vi "Show Cursors.vi"(6 "Cursor Options":T1={"font"={"Font Name"="Arial", "Size"=14, "Strikeout?"=FALSE, "Italic?"=FALSE, "Underline?"=FALSE, "Outline?"=FALSE, "Shadow?"=FALSE, "Bold?"=FALSE}, "size"=1, "Timestamp"=enum."at TOP", "Vertical Line?"=FALSE, "Horizontal Line?"=FALSE, "alignment(left, top)"={"horizontal"=enum."center", "vertical"=enum."center"}, "TextFormat"="%2$.2f\\n\\n%1$s", "time format (%H:%M:%S)"="Arial"} {"size" min=1 max=50}, 8 "error in (no error)":errorcluster, 9 "Coords":T2, 10 "XY Graph":refnum<vi>, 11 "input picture":picture) -> (0 "error out":errorcluster, 3 "output picture":picture)   [LabVIEW 2015]
doc: "Shows real time cursors overlayed in a graph, using just one mouse move event case. The options for the cursors can be highly customized to set up a unique cursor style.\n\nUsage: Place this inside an event structure on any XY graph, in the \"Mouse Move\" event case. Set the options as an input cluster to override the defaults. The output picture control would typically be connected to the XY Graph's \"PlotImages.Front\" property item.\n\nCursor Options\n<b>Horizontal Line?</b> - Draws a horizontal line to intersect each plot\n<b>Verticle Line?</b> - Draws a verticle line at the mouse location to highlight the cursor location (typically on the time scale)\n<b>Timestamp</b> - Sets where to display the timestamp (if you want it at the top or bottom) Used best with the verticle line turned on.\n<b>Font</b> - Setup the font for displaying the cursor text\n<b>Alignment</b> - Sets the alignment options for the text relative to the cursor point\n<b>TextFormat</b> - Sets the text display format at the cursor points to show. Three input parameters are available for the text, which can be accessed using parameter numbers.\ninputs: \n1$ - Timestamp at cursor locations\n2$ - Value of the plot\n3$ - Name of the plot\n\nExamples: $2$.2f\\n\\n%1$s\nThis shows the value of the plot with 2 decimal places. A blank line, then the name of the plot"
uses:
  <vilib>/Utility/miscctls.llb/LVPoint32TypeDef.ctl
  controls/CursorOptions.ctl
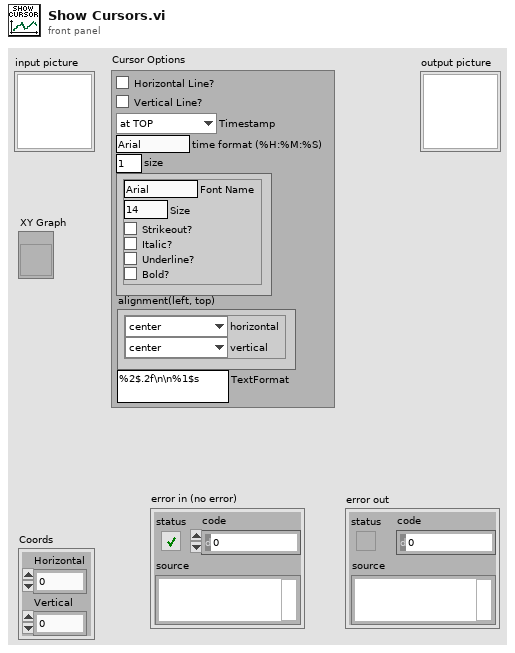
[diagram p1: front panel]
types:
  T1 = typedef "CursorOptions.ctl" = cluster{"font":cluster{"Font Name":string, "Size":i16, "Strikeout?":bool, "Italic?":bool, "Underline?":bool, "Outline?":bool, "Shadow?":bool, "Bold?":bool}, "size":i16, "Timestamp":enum16{"at TOP", "at BOTTOM", "none"}, "Vertical Line?":bool, "Horizontal Line?":bool, "alignment(left, top)":cluster{"horizontal":enum16{"left", "center", "right"}, "vertical":enum16{"top", "center", "bottom"}}, "TextFormat":string, "time format (%H:%M:%S)":string}
  T2 = typedef "LVPoint32TypeDef.ctl" = cluster{"Horizontal":i32, "Vertical":i32}
  T3 = enum16{"User-specified Font", "Application Font", "System Font", "Dialog Font"}
  T4 = cluster{"horizontal":enum16{"left", "center", "right"}, "vertical":enum16{"top", "center", "bottom"}}
  T5 = cluster{"Font Name":string, "Size":i16, "Strikeout?":bool, "Italic?":bool, "Underline?":bool, "Outline?":bool, "Shadow?":bool, "Bold?":bool}
  T6 = typedef "LVRectTypeDef.ctl" = cluster{"Left":i16, "Top":i16, "Right":i16, "Bottom":i16}
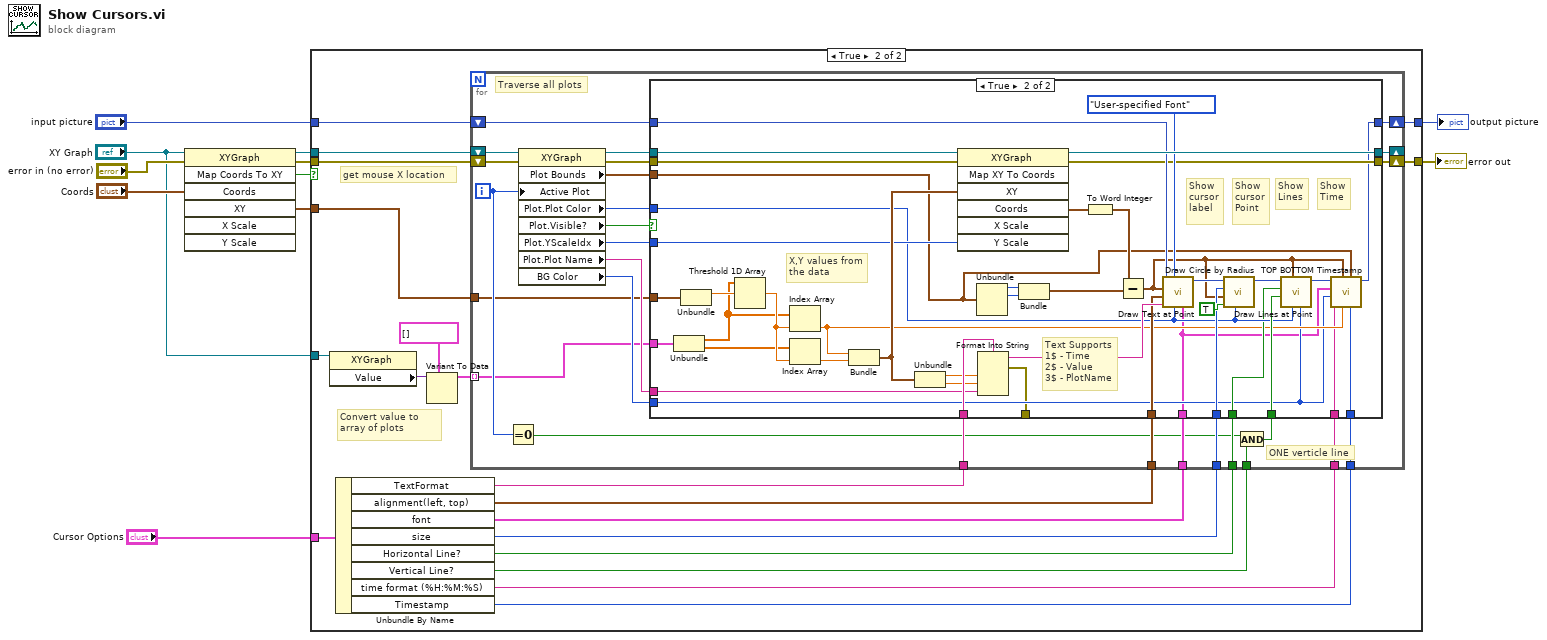
[diagram p0: block diagram]
diagram:
  n1 = invoke on="Invoke Node" class="XYGraph" method="Map Coords To XY"(reference="XY Graph", error in="error in (no error)", "Coords"="Coords") -> (reference out=w8:refnum<vi>, error out=w7:errorcluster, "Map Coords To XY"=w10:bool, "XY"=w11:cluster{"X":dbl, "Y":dbl})  [unwired: 4 in, 3 out]
  n2 = case shown="True" w10 {
    tunnel: w11 -> [_ w31]
    tunnel: w8 -> [_ w32]
    tunnel: [w12 w30] -> w3
    tunnel: w7 -> [w13 w29]
    tunnel: [w13 w28] -> w6
    tunnel: "input picture" -> [w12 w27]
    tunnel: "Cursor Options" -> [_ w19]
    tunnel: "XY Graph" -> [_ w16]
    frame False {
      # "not in plot area.  clear the image"
    }
    frame True {
      # "Convert value to array of plots"
      # "get mouse X location"
      n3 = property class="XYGraph"(reference=w16) -> ("Value"=w15:variant)  [unwired: 1 in, 2 out]
      n4 = Unbundle By Name(w19) -> ("TextFormat"=w26:string, "alignment(left, top)"=w25:T4, "font"=w24:T5, "size"=w23:i16, "Horizontal Line?"=w22:bool, "Vertical Line?"=w21:bool, "time format (%H:%M:%S)"=w14:string, "Timestamp"=w20:enum16{"at TOP", "at BOTTOM", "none"})
      n5 = Variant To Data(type=cluster{dbl[], dbl[]}[] [], Variant=w15) -> (data=w18:cluster{dbl[], dbl[]}[])  [unwired: 1 in, 1 out]
      n6 = for {
        tunnel: w18 -> [w34] mode=indexing
        shift-right: [w58] -> _
        shift-left: w32 -> [w56]
        tunnel: w31 -> [w35]
        shift-right: [w54] -> w30
        shift-left: w27 -> [w57]
        shift-right: [w49] -> w28
        shift-left: w29 -> [w51]
        tunnel: w23 -> [w47]
        tunnel: w25 -> [w46]
        tunnel: w24 -> [w45]
        tunnel: w26 -> [w44]
        tunnel: w22 -> [w43]
        tunnel: w21 -> [w39]
        tunnel: w20 -> [w37]
        tunnel: w14 -> [w33]
        i -> [w42]
        # "Traverse all plots"
        # "ONE verticle line"
        n7 = Equal To 0?(x=w42) -> (x = 0?=w40:bool)
        n8 = property on="Property Node" class="XYGraph"(reference=w56, error in=w51, "Active Plot"=w42) -> (reference out=w55:refnum<vi>, error out=w50:errorcluster, "Plot Bounds"=w59:T6, "Plot.Plot Color"=w53:u32, "Plot.Visible?"=w52:bool, "Plot.YScaleIdx"=w48:u32, "Plot.Plot Name"=w38:string, "BG Color"=w36:u32)
        n9 = And(x=w40, y=w39) -> (x .and. y?=w41:bool)
        n10 = case shown="True" w52 {
          tunnel: w59 -> [_ w68]
          tunnel: [w62 w100] -> w58
          tunnel: w34 -> [_ w95]
          tunnel: w35 -> [_ w94]
          tunnel: w57 -> [w61 w93]
          tunnel: w55 -> [w62 w90]
          tunnel: [w61 w73] -> w54
          tunnel: w53 -> [_ w78]
          tunnel: w50 -> [w60 w86]
          tunnel: [w60 w85] -> w49
          tunnel: w48 -> [_ w84]
          tunnel: w47 -> [_ w83]
          tunnel: w46 -> [_ w82]
          tunnel: w45 -> [_ w66]
          tunnel: w44 -> [_ w81]
          tunnel: w43 -> [_ w77]
          tunnel: w41 -> [_ w80]
          tunnel: w38 -> [_ w74]
          tunnel: w37 -> [_ w70]
          tunnel: w36 -> [_ w67]
          tunnel: [_ w64] -> _
          tunnel: w33 -> [_ w63]
          frame False {
            # "plot is not visible, so don't show the cursor for it."
          }
          frame True {
            # "Show\nTime"
            # "Show\nLines"
            # "Show\ncursor\nPoint"
            # "Show\ncursor\nlabel"
            # "Text Supports\n1$ - Time\n2$ - Value\n3$ - PlotName"
            # "X,Y values from the data"
            n11 = Unbundle(w95) -> (w65:dbl[], w97:dbl[])
            n12 = Unbundle(w94) -> ("X"=w96:dbl)  [unwired: 1 out]
            n13 = Threshold 1D Array(2:w96, 3:w65) -> (0:w98:dbl)  [unwired: 1 in]
            n14 = Index Array(array=w65, index=w98) -> (element=w71:dbl)
            n15 = Index Array(array=w97, index=w98) -> (element=w99:dbl)
            n16 = Bundle("X"=w71, "X"=w99) -> (w92:cluster{"X":dbl, "X":dbl})  [unwired: 1 in]
            n17 = Unbundle(w92) -> ("X"=w76:dbl, "X"=w75:dbl)
            n18 = invoke on="Invoke Node" class="XYGraph" method="Map XY To Coords"(reference=w90, error in=w86, "XY"=w92, "Y Scale"=w84) -> (reference out=w100:refnum<vi>, error out=w85:errorcluster, "Coords"=w105:T2)  [unwired: 3 in, 4 out]
            n19 = Unbundle(w68) -> ("Left"=w103:i16, "Top"=w104:i16)  [unwired: 2 out]
            n20 = Format Into String(format string=w81, w76, w75, w74) -> (resulting string=w91:string, error out=w64:errorcluster)  [unwired: 2 in]
            n21 = Bundle("Left"=w103, "Top"=w104) -> (w101:cluster{"Left":i16, "Top":i16})  [unwired: 1 in]
            n22 = To Word Integer(number=w105) -> (16bit integer=w102:cluster{"Horizontal":i16, "Vertical":i16})
            n23 = Subtract(x=w102, y=w101) -> (x-y=w69:cluster{i16, i16})
            n24 = call <vilib>:"Draw Text at Point.vi"("[user-specified font]"=w66, "text color(black)"=w78, "desired font(Application)"=T3."User-specified Font", "text"=w91, "alignment(left, top)"=w82, "origin"=w69, "picture"=w93) -> ("new picture"=w89:picture)  [unwired: 3 in, 1 out]
            n25 = call <vilib>:"Draw Circle by Radius.vi"("color(black)"=w78, "fill?(F)"=TRUE, "pixel center"=w69, "radius"=w83, "picture"=w89) -> ("new picture"=w79:picture)  [unwired: 6 in]
            n26 = call "Draw Lines at Point.vi"("GraphBGK"=w67, "color(black)"=w78, "pixel center"=w69, "Vertical Line?"=w80, "Horizontal Line?"=w77, "new picture in"=w79) -> ("new picture out"=w72:picture)  [unwired: 5 in]
            n27 = call "TOP BOTTOM Timestamp.vi"("Format"=w70, "Rect"=w68, "Timestamp"=w71, "pixel center"=w69, "time format (%H:%M:%S)"=w63, "GraphBGK"=w67, "font"=w66, "new picture in"=w72) -> ("new picture out"=w73:picture)  [unwired: 3 in]
          }
        }
      }
    }
  }
  "error out" <- w6
  "output picture" <- w3
